vi "PH_Sequencer.PC _6P_4Q_Pos.vi"(0 "VI in":refnum<vi>, 2 "Selector":T1 items=["unknown", "Position I", "Position II", "Position III", "Position IV", "moving"], 3 "serviceName":string, 4 "linked?":bool, 5 "error in":errorcluster) -> (14 "VI out":refnum<vi>, 19 "error out":errorcluster)   [LabVIEW 2014, in "PH_Sequencer.lvlib"]
doc: "This VI stores information at own attributes and forces some action at first linkage."
uses:
  PH_Sequencer.lvlib
  PH_4_Pos_Selector/PH_4_Pos_Selector.Position Selector.ctl
  PH_Beamline/PH_Beamline.6P 4 Pos Selector Instances.ctl
  PH_Beamline/PH_Beamline.lvlib
  PH_BeamlineInformation/PH_BeamlineInformation.lvlib
  PH_4_Pos_Selector/PH_4_Pos_Selector.lvlib
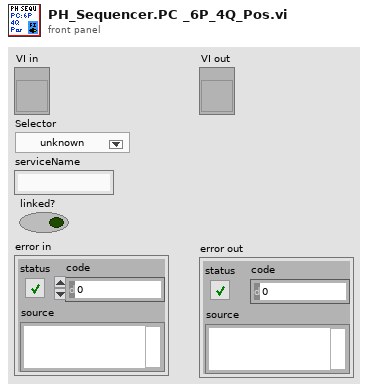
[diagram p1: front panel]
types:
  T1 = typedef "PH_4_Pos_Selector.lvlib/PH_4_Pos_Selector.Position Selector.ctl" = u16
  T2 = typedef "PH_Sequencer.lvlib/PH_Sequencer.i attribute.ctl" = cluster{"GUI Refs":cluster{"Main Off":refnum<vi>, "Fire":refnum<vi>, "Status":refnum<vi>, "Ready":refnum<vi>, "Waiting Time":refnum<vi>, "Timeout":refnum<vi>, "PPMA Ready":refnum<vi>, "Sequencer SM State":refnum<vi>, "PPPA Ready":refnum<vi>, "Calorimeter":refnum<vi>, "Beamline Ready":refnum<vi>, "Clear Beamline":refnum<vi>, "Linkage PPMA Rods":refnum<vi>, "Linkage Current PA":refnum<vi>, "Linkage Current MA":refnum<vi>, "Timing Ready":refnum<vi>, "State Timing":refnum<vi>, "Force Timing":refnum<vi>, "PSDB Shot Comment":refnum<vi>, "State PA Backreflection":refnum<vi>, "Beamline Z6 Ready":refnum<vi>, "Clear Z6 Beamline":refnum<vi>, "Sequence length":refnum<vi>, "Timing Mode":refnum<vi>, "Slow Trigger Settings":refnum<vi>, "Experiment Description":refnum<vi>, "State PSDB":refnum<vi>, "PSDB Ready":refnum<vi>, "Set PSDB Settings":refnum<vi>, "Get PSDB Info":refnum<vi>, "Take Snapshot":refnum<vi>, "Shottype":refnum<vi>, "Experiment":refnum<vi>, "Phase Frontends":refnum<vi>, "PP 45mm PILC in use":refnum<vi>}, "Status Info":cluster{"Machine Status":T3, "WaitingTime":i32, "Timeout":bool}, "Readyness":cluster{"Ready to shot":bool, "PPMA Ready":bool, "PPPA Ready":bool, "BL Ready":bool, "Timing Ready":bool, "BL Z6 Ready":bool, "PSDBReady":bool}, "Instancenames":cluster{"PPMA Rods":string, "PP Current Meas":string, "PH Beamline Chief":string, "PA Backrefl Meas":string, "Z6 Beamline Chief":string}, "Data to read":bool, "Calorimeter":cluster{"Instancename":string, "On":bool, "linked":bool}, "Linkage":cluster{"PPMA Rods":bool, "PP Current Meas":bool, "PHELIX Beamline Chief":bool, "PA Backrefl Meas":bool, "Z6 Beamline Chief":bool}, "Timing":cluster{"Instance":string, "linked":bool, "Status":T3, "Timing Mode":T4, "Slow Trigger Settings":T5, "Info available":cluster{"ext SlowTrigger":bool, "T2":bool, "Mode":bool, "Delay Slow Trigger":bool, "Phase FEs":bool}, "FE Phase":T6}, "Service ID R2S":i32, "PSDB":cluster{"Controller Instance":string, "Controller Status":T3, "Controller linked":bool, "Settings acknowledged":bool, "Current Experiment ID":i16, "Current Shot Type":i16, "Current Comment":string, "Remember Settings":bool, "Write 2 early":bool}, "PSDB Data":cluster{"Main Off?":bool, "Sequence Length":dbl, "Sequence startet":timestamp}, "6P 4Q Positions":cluster{"Instancename":string, "linked":bool, "Position":T1}[], "PUs":T7[]}
  T3 = typedef "PH_StatusHandler.lvlib/PH_StatusHandler.Status.ctl" = i16
  T4 = typedef "PH_Timing.lvlib/PH_Timing.Timing Mode.ctl" = cluster{"T2":i16, "Modeselector":enum32{"10 Hz", "0.5 Hz", "Shot"}}
  T5 = typedef "PH_Timing.lvlib/PH_Timing.Slow Trigger Settings.ctl" = cluster{"Delay":dbl, "externally triggered?":bool}
  T6 = typedef "PH_Timing.lvlib/PH_Timing.Phase FEs.ctl" = cluster{"Phase":dbl}
  T7 = typedef "PH_Sequencer.lvlib/PH_Sequencer.Head.ctl" = cluster{"PowerUnit":T8, "GUI Ref":refnum<vi>, "Information":T9, "linked?":bool, "GUI Ref Current Voltage":refnum<vi>}
  T8 = typedef "PH_PP_Common.lvlib/PH_PP_Common.PUs.ctl" = enum16{"no Info", "PA-19mm-1", "PA-19mm-2", "PA-45mm-PILC", "PA-45mm-MAIN", "MA-PU-1", "MA-PU-2", "MA-PU-3", "MA-PU-4", "MA-PU-5", "MA-PU-6", "MA-FR", "MA-PILC", "PA-45mm-DP"}
  T9 = typedef "PH_Sequencer.lvlib/PH_Sequencer.PU Information.ctl" = cluster{"State":T3, "Waiting Time [s]":dbl, "PU State SM":T10, "PU Timeout SM":T10}
  T10 = typedef "PH_PowerUnit_BaseClass.lvlib/PH_PowerUnit_BaseClass.SM States.ctl" = enum16{".", "Stand by", "Switch PU on", "Configure", "Set Default Voltage", "Set STANDBY", "Set READY", "Wait for Shot Cmd", "Open Dump Rods", "Open Ross Relais", "Close Ross Relais", "Switch PSU on", "Switch PSU off", "Charge", "Switch GD Channel on", "Close Dump Rods", "Rods-TO", "RR-TO", "PSU-TO", "Trigger-TO"}
  T11 = typedef "PH_Beamline.lvlib/PH_Beamline.6P 4 Pos Selector Instances.ctl" = string
  T12 = cluster{"Instancename":string, "linked":bool, "Position":T1}[]
  T13 = cluster{"Instancename":string, "linked":bool, "Position":T1}
  T14 = typedef "PH_BeamlineInformation.lvlib/PH_BeamlineInformation.i attribute.ctl" = cluster{"BL GUI Elements of Services":cluster{"Service Name":string, "GUI Elements":refnum<vi>[], "Status":i32}[], "Powermeters":T15, "Efficiency":T16, "Heads":T17[]}
  T15 = typedef "PH_BeamlineInformation.lvlib/PH_BeamlineInformation.Powermeter.ctl" = cluster{"ns FE":cluster{"GUI Ref":refnum<vi>, "Value":dbl}, "fs FE":cluster{"GUI Ref":refnum<vi>, "Value":dbl}, "PA":cluster{"GUI Ref":refnum<vi>, "Value":dbl}, "MA":cluster{"GUI Ref":refnum<vi>, "Value":dbl}, "Z6 green":cluster{"GUI Ref":refnum<vi>, "Value":dbl}, "Z6 IR":cluster{"GUI Ref":refnum<vi>, "Value":dbl}, "Z6 COS":cluster{"GUI Ref":refnum<vi>, "Value":dbl}}
  T16 = typedef "PH_BeamlineInformation.lvlib/PH_BeamlineInformation.Efficiency.ctl" = cluster{"PA Gain":cluster{"GUI Ref":refnum<vi>, "Value":dbl}, "MA Gain":cluster{"GUI Ref":refnum<vi>, "Value":dbl}, "Z6 green Conversion":cluster{"GUI Ref":refnum<vi>, "Value":dbl}, "Z6 Comp Losses":cluster{"GUI Ref":refnum<vi>, "Value":dbl}}
  T17 = typedef "PH_BeamlineInformation.lvlib/PH_BeamlineInformation.Head.ctl" = cluster{"PowerUnit":T8, "in use":cluster{"Value":bool, "GUI Ref":refnum<vi>, "linked":bool}, "voltage":cluster{"Value":dbl, "GUI Ref":refnum<vi>, "linked":bool}}
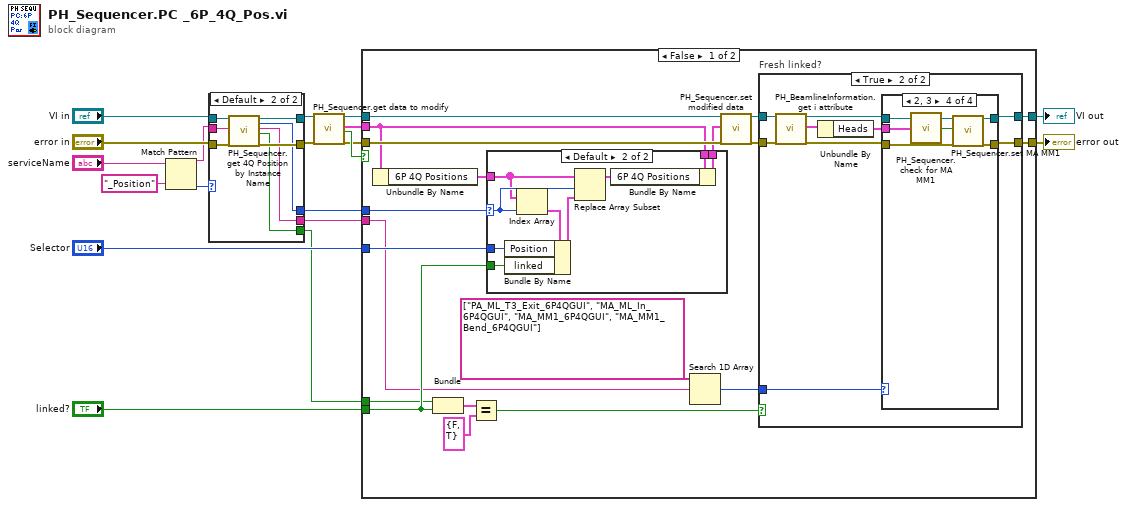
[diagram p0: block diagram]
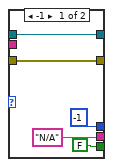
[diagram p2: hidden frame]
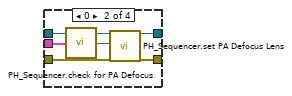
[diagram p5: hidden frame]
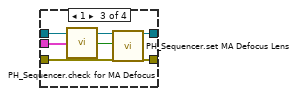
[diagram p6: hidden frame]
diagram:
  n1 = Match Pattern(string="serviceName", regular expression="_Position" ("string")) -> (before substring=w5:string, offset past match=w4:i32)  [unwired: 1 in, 2 out]
  n2 = case shown="Default" w4 {
    tunnel: "error in" -> [w23 w32]
    tunnel: [w23 w31] -> w10
    tunnel: "VI in" -> [w24 w30]
    tunnel: [w24 w29] -> w8
    tunnel: w5 -> [_ w28]
    tunnel: [-1 ("index of element") w27] -> w3
    tunnel: [FALSE ("linked") w26] -> w2
    tunnel: ["N/A" ("Instancename") w25] -> w1
    frame -1 {
    }
    frame Default {
      n3 = call "PH_Sequencer.get 4Q Position by Instance Name.vi"("VI in"=w30, "Wanted 4Q Instance"=w28, "error in"=w32) -> ("VI out"=w29:refnum<vi>, "index of element"=w27:i32, "Instancename"=w25:string, "linked"=w26:bool, "error out"=w31:errorcluster)  [unwired: 11 in, 1 out]
    }
  }
  n4 = call "PH_Sequencer.get data to modify.vi"("i ref in"=w8, "error in (no error)"=w10) -> ("i ref out"=w15:refnum<vi>, "i attribute"=w18:T2, "timed out"=w17:bool, "error out"=w12:errorcluster)  [unwired: 14 in]
  n5 = case shown="False" w17 {
    tunnel: w12 -> [w51 w93]
    tunnel: "Selector" -> [w45 _]
    tunnel: [w44 w93] -> w14
    tunnel: w15 -> [w50 w94]
    tunnel: [w42 w94] -> w16
    tunnel: w18 -> [w48 _]
    tunnel: "linked?" -> [w41 _]
    tunnel: w3 -> [w33 _]
    tunnel: w2 -> [w37 _]
    tunnel: w1 -> [w36 _]
    frame False {
      n6 = Unbundle By Name(w48) -> ("6P 4Q Positions"=w46:T12)
      n7 = Bundle("linked"=w37, "linked?"=w41) -> (w40:cluster{"linked":bool, "linked?":bool})  [unwired: 1 in]
      n8 = Equal?(x=w40, y=cluster{"linked":bool, "linked?":bool} {"linked"=FALSE, "linked?"=TRUE}) -> (x = y?=w38:bool)
      n9 = case shown="Default" w33 {
        selector: w33 -> [_ w86]
        tunnel: [w83 w92] -> w49
        tunnel: w48 -> [w83 w91]
        tunnel: w46 -> [_ w85]
        tunnel: w45 -> [_ w88]
        tunnel: w41 -> [_ w87]
        frame -1 {
        }
        frame Default {
          n10 = Index Array(array=w85, index=w86) -> (element=w84:T13)
          n11 = Bundle By Name(cluster=w84, "Position"=w88, "linked"=w87) -> (w89:T13)
          n12 = Replace Array Subset(array=w85, new element=w89, index=w86) -> (w90:T12)
          n13 = Bundle By Name(cluster=w91, "6P 4Q Positions"=w90) -> (w92:T2)
        }
      }
      n14 = Search 1D Array(1D array=T11[] ["PA_ML_T3_Exit_6P4QGUI", "MA_ML_In_6P4QGUI", "MA_MM1_6P4QGUI", "MA_MM1_Bend_6P4QGUI"], element=w36) -> (index of element=w34:i32)  [unwired: 1 in]
      n15 = call "PH_Sequencer.set modified data.vi"("i ref in"=w50, "i attribute"=w49, "error in (no error)"=w51) -> ("i ref out"=w43:refnum<vi>, "error out"=w47:errorcluster)  [unwired: 15 in]
      n16 = case "Fresh linked?" shown="True" w38 {
        tunnel: w47 -> [w52 w57]
        tunnel: [w52 w62] -> w44
        tunnel: w43 -> [w53 w59]
        tunnel: [w53 w61] -> w42
        tunnel: w34 -> [_ w60]
        frame False {
        }
        frame True {
          n17 = call "PH_BeamlineInformation.get i attribute.vi"("i ref in"=w59, "error in (no error)"=w57) -> ("i ref out"=w58:refnum<vi>, "i attribute"=w55:T14, "error out"=w56:errorcluster)  [unwired: 15 in]
          n18 = Unbundle By Name(w55) -> ("Heads"=w54:T17[])
          n19 = case shown="2, 3" w60 {
            tunnel: w56 -> [w63 w70 w76 w82]
            tunnel: [w63 w69 w75 w81] -> w62
            tunnel: w58 -> [w64 w68 w74 w80]
            tunnel: [w64 w67 w73 w79] -> w61
            tunnel: w54 -> [_ w66 w72 w78]
            frame Default {
            }
            frame 0 {
              n20 = call "PH_Sequencer.check for PA Defocus.vi"("Heads"=w66) -> ("PA Defocus must be set?"=w65:bool)
              n21 = call "PH_Sequencer.set PA Defocus Lens.vi"("i ref in"=w68, "Shotposition?"=w65, "error in"=w70) -> ("i ref out"=w67:refnum<vi>, "error out"=w69:errorcluster)  [unwired: 15 in]
            }
            frame 1 {
              n22 = call "PH_Sequencer.check for MA Defocus.vi"("Heads"=w72) -> ("MA Defocus must be set?"=w71:bool)
              n23 = call "PH_Sequencer.set MA Defocus Lens.vi"("i ref in"=w74, "Shotposition?"=w71, "error in"=w76) -> ("i ref out"=w73:refnum<vi>, "error out"=w75:errorcluster)  [unwired: 15 in]
            }
            frame 2, 3 {
              n24 = call "PH_Sequencer.check for MA MM1.vi"("Heads"=w78) -> ("MA MM1 must be set?"=w77:bool)
              n25 = call "PH_Sequencer.set MA MM1.vi"("i ref in"=w80, "High Energy Position?"=w77, "error in"=w82) -> ("i ref out"=w79:refnum<vi>, "error out"=w81:errorcluster)  [unwired: 15 in]
            }
          }
        }
      }
    }
    frame True {
    }
  }
  "VI out" <- w16
  "error out" <- w14
